vi "Get BLISS_files with valid extensions.vi"(8 "error in (no error)":errorcluster, 9 "extensions":string[](array[string]), 11 "path in":path) -> (0 "error out":errorcluster, 2 "valid filepaths":path[](array[path]), 3 "valid files":string[](array[string]))   [LabVIEW 2020]
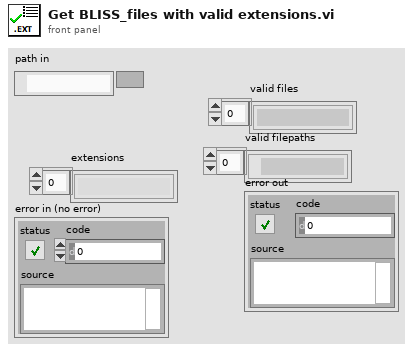
[diagram p1: front panel]
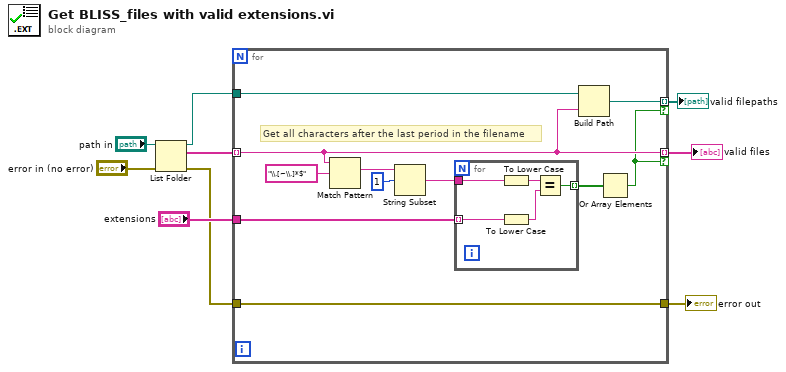
[diagram p0: block diagram]
diagram:
  n1 = List Folder(path="path in", error in="error in (no error)") -> (path out=w5:path, filenames=w7:string[], error out=w3:errorcluster)  [unwired: 2 in, 1 out]
  n2 = for {
    tunnel: w7 -> [w13] mode=indexing
    tunnel: [w13] -> w8 mode=indexing if=w11
    tunnel: "extensions" -> [w15]
    tunnel: w5 -> [w14]
    tunnel: [w12] -> w4 mode=indexing if=w11
    tunnel: w3 -> [w10]
    tunnel: [w10] -> w2
    # "Get all characters after the last period in the filename"
    n3 = Match Pattern(string=w13, regular expression="\\.[~\\.]*$") -> (match substring=w19:string)  [unwired: 4 out]
    n4 = String Subset(string=w19, offset (0)=1) -> (substring=w20:string)  [unwired: 1 out]
    n5 = for {
      tunnel: w20 -> [w25]
      tunnel: [w22] -> w16 mode=indexing
      tunnel: w15 -> [w21] mode=indexing
      n6 = To Lower Case(string=w25) -> (all lower case string=w24:string)
      n7 = To Lower Case(string=w21) -> (all lower case string=w23:string)
      n8 = Equal?(x=w24, y=w23) -> (x = y?=w22:bool)
    }
    n9 = Build Path(base path=w14, name or relative path=w13) -> (appended path=w12:path)
    n10 = Or Array Elements(Boolean array=w16) -> (logical OR=w11:bool)
  }
  "valid files" <- w8
  "valid filepaths" <- w4
  "error out" <- w2
